vi "setfracLUT.vi"(1 "Frequency":dbl=1000.0, 2 "Number of entries in LUT":dbl=2000.0, 3 "Input":dbl) -> (0 "Fraction":dbl)   [LabVIEW 2012]
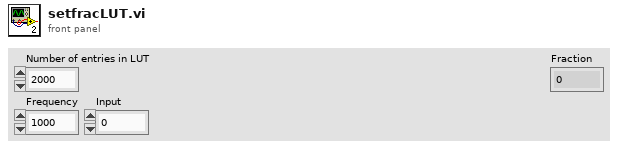
[diagram p1: front panel]
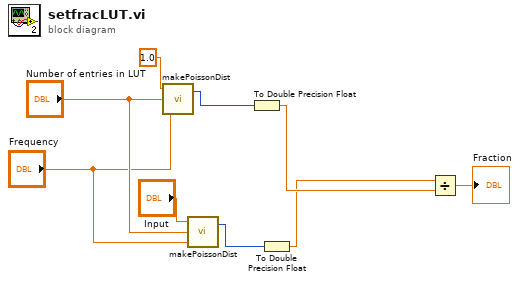
[diagram p0: block diagram]
diagram:
  n1 = call "makePoissonDist.vi"("Frequency"="Frequency", "Number of entries in LUT"="Number of entries in LUT", "Input"=1.0) -> ("Output"=w8:u32)  [unwired: 1 out]
  n2 = call "makePoissonDist.vi"("Frequency"="Frequency", "Number of entries in LUT"="Number of entries in LUT", "Input"="Input") -> ("Output"=w4:u32)  [unwired: 1 out]
  n3 = To Double Precision Float(number=w8) -> (double precision float=w2:dbl)
  n4 = To Double Precision Float(number=w4) -> (double precision float=w1:dbl)
  n5 = Divide(x=w1, y=w2) -> (x/y=→"Fraction":dbl)
